vi "TurnDegrees to MM Setpoints.vi"(2 "Turn Degrees":dbl) -> (0 "Right MM Setpoint":dbl, 1 "Left MM Setpoint":dbl)   [LabVIEW 2018]
panel:
  in  "Track Width":dbl
  # "CURRENTLY STUB VI\n\nNot anymore because of us."
  # "Will Need to create some \nnumbers for trig in constants.vi\nFor example: Trackwidth\n\n\n\n\n\n\n\n\n\n\n\n\n\n\n\n\n\nProduct of Cyril Ng and Hermela Benyam"
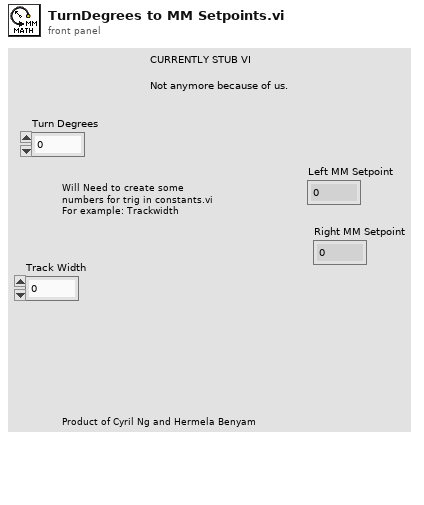
[diagram p1: front panel]
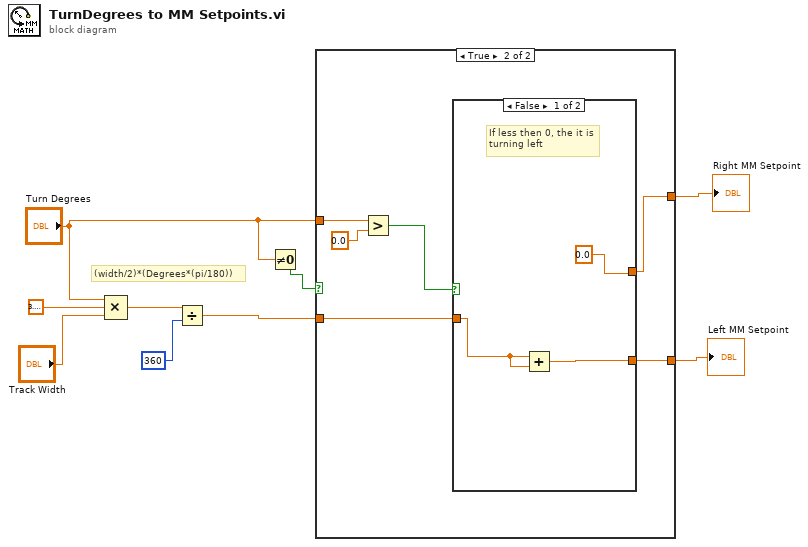
[diagram p0: block diagram]
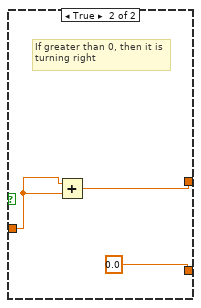
[diagram p3: hidden frame]
diagram:
  # "(width/2)*(Degrees*(pi/180))"
  n1 = Compound Arithmetic op=MULTIPLY("Turn Degrees", 3.141592653589793, "Track Width") -> (w6:dbl)
  n2 = Divide(x=w6, y=360) -> (x/y=w5:dbl)
  n3 = Not Equal To 0?(x="Turn Degrees") -> (x != 0?=w1:bool)
  n4 = case shown="True" w1 {
    tunnel: "Turn Degrees" -> [_ w15]
    tunnel: w5 -> [w10 w13]
    tunnel: [w10 w12] -> w4
    tunnel: [w10 w11] -> w3
    frame False {
    }
    frame True {
      n5 = Greater?(x=w15, y=0.0) -> (0:w14:bool)
      n6 = case shown="False" w14 {
        tunnel: w13 -> [w19 w22]
        tunnel: [0.0 w20] -> w11
        tunnel: [w17 0.0] -> w12
        frame False {
          # "If less then 0, the it is\nturning left"
          n7 = Add(x=w19, y=w19) -> (x+y=w17:dbl)
        }
        frame True {
          # "If greater than 0, then it is\nturning right"
          n8 = Add(x=w22, y=w22) -> (x+y=w20:dbl)
        }
      }
    }
  }
  "Right MM Setpoint" <- w3
  "Left MM Setpoint" <- w4
